vi "Save Image for Report.vi"(8 "error in (no error)":errorcluster, 10 "Test Image":picture, 11 "UUT Image":picture) -> (0 "error out":errorcluster, 3 "Image Report String":string)   [LabVIEW 2011]
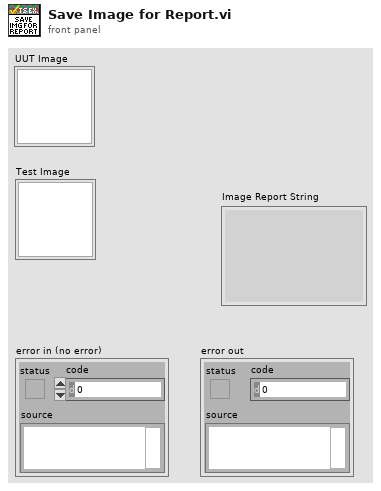
[diagram p1: front panel]
types:
  T1 = typedef "imagedata.ctl" = cluster{"image type":i32, "image depth":i32, "image":u8[], "mask":u8[], "colors":u32[], "Rectangle":cluster{"left":i16, "top":i16, "right":i16, "bottom":i16}}
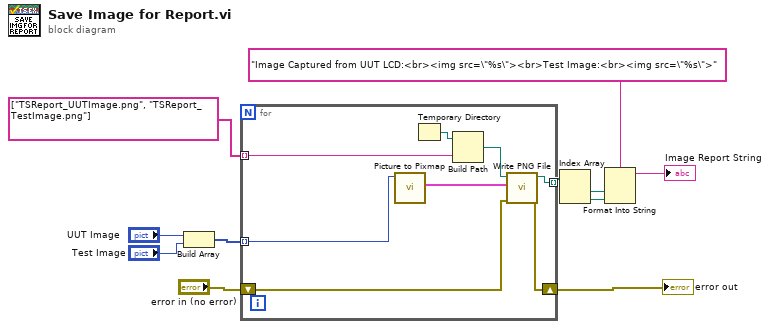
[diagram p0: block diagram]
diagram:
  n1 = Build Array("UUT Image", "Test Image") -> (w7:picture[])
  n2 = for {
    tunnel: [w16] -> w6 mode=indexing
    tunnel: w7 -> [w15] mode=indexing
    tunnel: string[] ["TSReport_UUTImage.png", "TSReport_TestImage.png"] -> [w14] mode=indexing
    shift-right: [w13] -> w1
    shift-left: "error in (no error)" -> [w12]
    n3 = call <vilib>:"Picture to Pixmap.vi"("picture"=w15) -> ("image data"=w18:T1)  [unwired: 9 in, 1 out]
    n4 = Temporary Directory() -> (w19:path)
    n5 = Build Path(base path=w19, name or relative path=w14) -> (appended path=w17:path)
    n6 = call <vilib>:"Write PNG File.vi"("error in (no error)"=w12, "image data"=w18, "path to PNG file"=w17) -> ("error out"=w13:errorcluster, "path"=w16:path)  [unwired: 7 in]
  }
  "error out" <- w1
  n7 = Index Array(array=w6) -> (element #1=w5:path, element #2=w4:path)  [unwired: 2 in]
  n8 = Format Into String(format string="Image Captured from UUT LCD:<br><img src=\"%s\"><br>Test Image:<br><img src=\"%s\">", w5, w4) -> (resulting string=→"Image Report String":string)  [unwired: 2 in, 1 out]
